vi "Configure Module.vi"(8 "error in (no error)":errorcluster, 10 "IOV ref in":variant, 11 "9213 in":refnum<class "9212.lvclass">) -> (0 "error out":errorcluster, 2 "IOV ref out":variant, 3 "9213 out":refnum<class "9212.lvclass">)   [LabVIEW 2020, in "Modules.lvlib" / "9212.lvclass"]
uses:
  9212.lvclass
  <resource>/objmgr/cRIO.rc
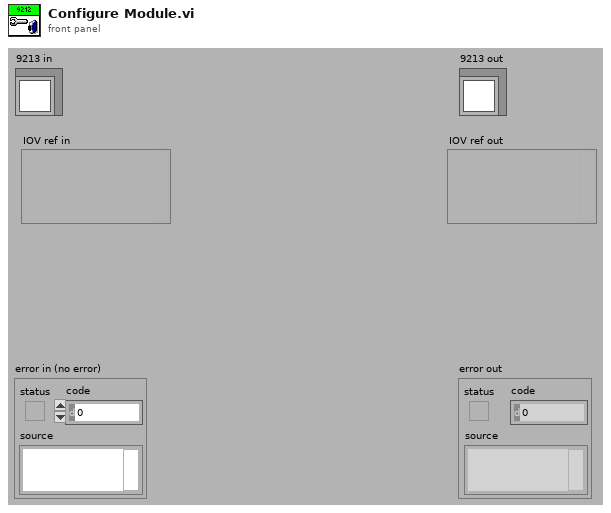
[diagram p1: front panel]
types:
  T1 = typedef "Modules.lvlib/9212.lvclass/Conversion Time.ctl" = u16
  T2 = typedef "Modules.lvlib/9212.lvclass/Measurement Units.ctl" = u8
  T3 = typedef "Modules.lvlib/9212.lvclass/Thermocouple Type.ctl" = u8
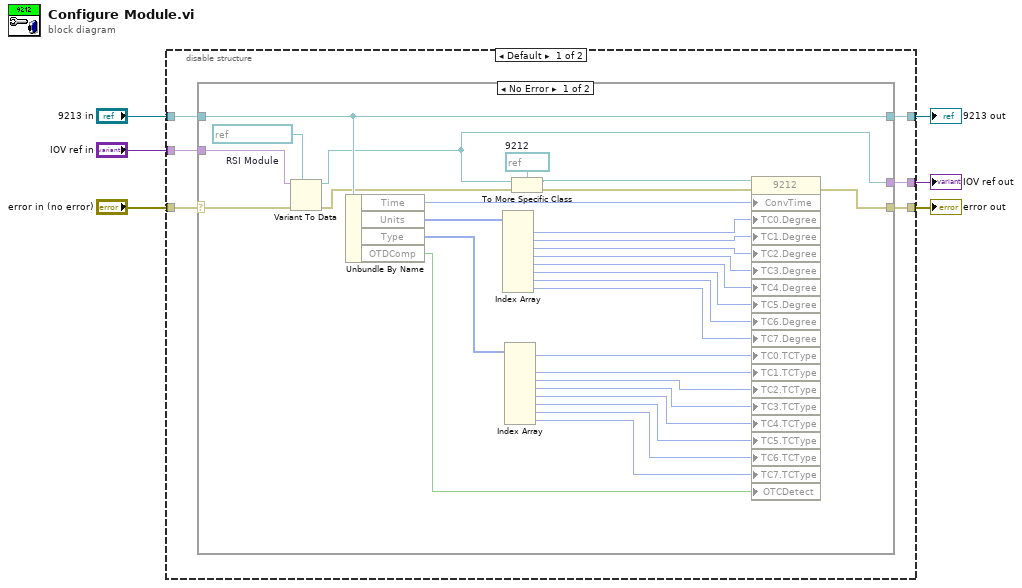
[diagram p0: block diagram]
diagram:
  n1 = disable-structure shown="Default" {
    disable-tunnel: "error in (no error)" -> [w12 w48]
    disable-tunnel: [w11 w48] -> w5
    disable-tunnel: "9213 in" -> [w10 w46]
    disable-tunnel: [w9 w46] -> w3
    disable-tunnel: "IOV ref in" -> [w8 w47]
    disable-tunnel: [w7 w47] -> w1
    frame condition #0 {
      n2 = case shown="No Error" w12 {
        selector: w12 -> [w39 w45]
        tunnel: [w42 w45] -> w11
        tunnel: [w18 w44] -> w9
        tunnel: w10 -> [w18 w44]
        tunnel: w8 -> [w15 w43]
        tunnel: [w14 w43] -> w7
        frame No Error {
          w13 = refnum<k21> refnum  # RSI Module
          w38 = refnum<k21> refnum  # 9212
          n3 = Variant To Data(error in=w39, type=w13, Variant=w15) -> (data=w14:refnum<k21>, error out=w16:errorcluster)
          n4 = Unbundle By Name(w18) -> ("Time"=w19:T1, "Units"=w41:T2[], "Type"=w40:T3[], "OTDComp"=w17:bool)
          n5 = Index Array(array=w41) -> (element #1=w35:T2, element #2=w34:T2, element #3=w33:T2, element #4=w32:T2, element #5=w31:T2, element #6=w30:T2, element #7=w29:T2, element #8=w28:T2)  [unwired: 8 in]
          n6 = Index Array(array=w40) -> (element #1=w27:T3, element #2=w26:T3, element #3=w25:T3, element #4=w24:T3, element #5=w23:T3, element #6=w22:T3, element #7=w21:T3, element #8=w20:T3)  [unwired: 8 in]
          n7 = To More Specific Class(target class=w38, reference=w14, error in=w16) -> (specific class reference=w37:refnum<k21>, error out=w36:errorcluster)
          n8 = property class="9212"(reference=w37, error in=w36, "ConvTime"=w19, "TC0.Degree"=w35, "TC1.Degree"=w34, "TC2.Degree"=w33, "TC3.Degree"=w32, "TC4.Degree"=w31, "TC5.Degree"=w30, "TC6.Degree"=w29, "TC7.Degree"=w28, "TC0.TCType"=w27, "TC1.TCType"=w26, "TC2.TCType"=w25, "TC3.TCType"=w24, "TC4.TCType"=w23, "TC5.TCType"=w22, "TC6.TCType"=w21, "TC7.TCType"=w20, "OTCDetect"=w17) -> (error out=w42:errorcluster)  [unwired: 1 out]
        }
        frame Error {
        }
      }
    }
    frame condition #1 (active) {
    }
  }
  "error out" <- w5
  "9213 out" <- w3
  "IOV ref out" <- w1
